vi "Calibrations_Save.vi"(8 "error in":errorcluster, 11 "Subsystem":string="MySubsystem") -> (0 "error out":errorcluster)   [LabVIEW 2020]
uses:
  <vilib>/Utility/config.llb/Write Key (I32).vi
  <vilib>/Rock Robotics/Network Tables/NT Write Number.vi
  <vilib>/Utility/config.llb/Write Key (Double).vi
  <vilib>/Rock Robotics/Network Tables/NT Write String.vi
  <vilib>/Utility/config.llb/Write Key (String).vi
  <vilib>/Utility/config.llb/Write Key (Boolean).vi
  <vilib>/Rock Robotics/Network Tables/NT Write Boolean.vi
  <vilib>/Utility/config.llb/NI_LVConfig.lvlib
  <vilib>/Utility/Data Type/NI_Data Type.lvlib
panel:
  # "The calling VI will need to include a reference for the subsystem Global.vi. If this is omitted, this VI will not\nbe able to resolve the reference to the VI to iterate through the front-panel controls.e"
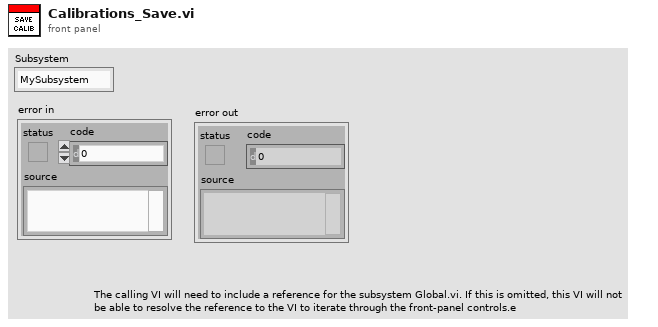
[diagram p1: front panel]
types:
  T1 = typedef "NI_LVConfig.lvlib/Config Data RefNum.ctl" = refnum<k1>
  T2 = typedef "NI_Data Type.lvlib/Data Type.ctl" = enum8{"Invalid Type", "Void", "I8", "I16", "I32", "I64", "U8", "U16", "U32", "U64", "Single Float", "Double Float", "Extended Float", "Single Complex", "Double Complex", "Extended Complex", "Enum U8", "Enum U16", "Enum U32", "Enum U64", "Single Float With Unit", "Double Float With Unit", "Extended Float With Unit", "Single Complex with Unit", "Double Complex with Unit", "Extended Complex with Unit", "Boolean", "String", "Path", "Picture", "Tag", "Array", "Cluster", "Variant", "LV Variant", "Waveform", "Timestamp", "Digital Waveform", "Digital Data", "ExpressData", "Refnum", "External Data", "VI", "Poly VI", "LabVIEW Class Instance", "Fixed Point", "Set Collection", "Map Collection"}
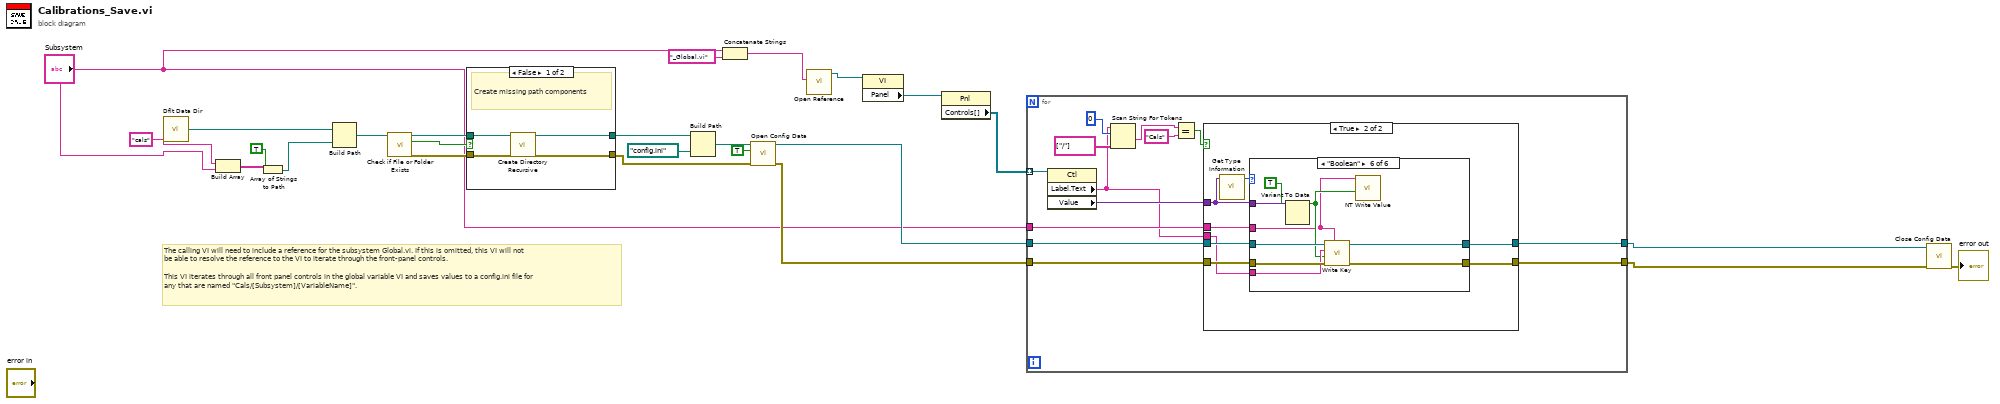
[diagram p0: block diagram]
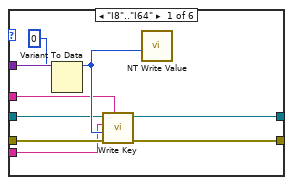
[diagram p3: hidden frame]
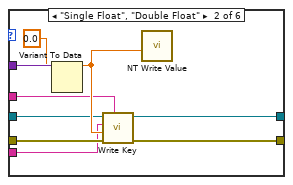
[diagram p4: hidden frame]
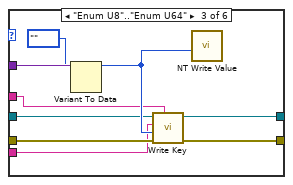
[diagram p5: hidden frame]
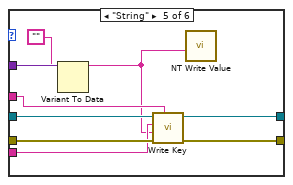
[diagram p7: hidden frame]
diagram:
  # "The calling VI will need to include a reference for the subsystem Global.vi. If this is omitted, this VI will not\nbe able to resolve the reference to the VI to iterate through the front-panel controls.\n\nThis VI iterates through all front panel controls in the global variable VI and saves values to a config.ini file for\nany that are named \"Cals/[Subsystem]/[VariableName]\"."
  n1 = call <vilib>:"Dflt Data Dir.vi"() -> ("App:Default Data Directory"=w25:path)
  n2 = Build Array("cals" ("string"), "Subsystem") -> (w4:string[])
  n3 = Array of Strings to Path(0:w4, 1:TRUE ("relative")) -> (2:w3:path)
  n4 = Build Path(base path=w25, name or relative path=w3) -> (appended path=w24:path)
  n5 = call <vilib>:"Check if File or Folder Exists.vi"("path"=w24) -> ("error out"=w21:errorcluster, "file or folder exists?"=w23:bool, "dup path"=w22:path)  [unwired: 8 in]
  n6 = case shown="False" w23 {
    tunnel: w22 -> [w29 w31]
    tunnel: w21 -> [w28 w30]
    tunnel: [w27 w31] -> w20
    tunnel: [w26 w30] -> w16
    frame False {
      # "Create missing path components"
      n7 = call <vilib>:"Create Directory Recursive.vi"("error in (no error)"=w28, "directory"=w29) -> ("error out"=w26:errorcluster, "directory copy"=w27:path)  [unwired: 3 in, 1 out]
    }
    frame True {
      # "Bypass"
    }
  }
  n8 = Build Path(base path=w20, name or relative path=path "config.ini") -> (appended path=w18:path)
  n9 = Concatenate Strings("Subsystem", "_Global.vi" ("string")) -> (w14:string)
  n10 = call <vilib>:"Open Config Data.vi"("error in (no error)"=w16, "create file if necessary (T)"=TRUE, "configuration file path"=w18) -> ("error out"=w7:errorcluster, "refnum"=w10:T1)  [unwired: 6 in, 1 out]
  n11 = call "Open Reference.vi"("Front Panel VI Name"=w14) -> ("Front Panel Reference"=w13:refnum<vi>)  [unwired: 5 in, 1 out]
  n12 = property class="VI"(reference=w13) -> ("Panel"=w12:refnum<vi>)  [unwired: 1 in, 2 out]
  n13 = property class="Pnl"(reference=w12) -> ("Controls[]"=w11:refnum<vi>[])  [unwired: 1 in, 2 out]
  n14 = for {
    tunnel: w11 -> [w44] mode=indexing
    tunnel: w10 -> [w42]
    tunnel: "Subsystem" -> [w41]
    tunnel: [w40] -> w9
    tunnel: [w39] -> w8
    tunnel: w7 -> [w38]
    n15 = property class="Ctl"(reference=w44) -> ("Label.Text"=w33:string, "Value"=w43:variant)  [unwired: 1 in, 2 out]
    n16 = Scan String For Tokens(6:string[] ["/"] ("operators (none)"), 8:0 ("offset"), 9:w33) -> (1:w32:string)  [unwired: 3 in, 3 out]
    n17 = Equal?(x=w32, y="Cals") -> (x = y?=w34:bool)
    n18 = case shown="True" w34 {
      tunnel: w43 -> [_ w53]
      tunnel: w42 -> [w46 w52]
      tunnel: w41 -> [_ w51]
      tunnel: [w46 w50] -> w40
      tunnel: [w45 w49] -> w39
      tunnel: w38 -> [w45 w48]
      tunnel: w33 -> [_ w47]
      frame False {
      }
      frame True {
        n19 = call <vilib>:"Get Type Information.vi"("variant"=w53) -> ("type"=w54:T2)  [unwired: 6 in, 4 out]
        n20 = case shown="\"Boolean\"" w54 {
          tunnel: w53 -> [w63 w72 w81 _ w86 w96]
          tunnel: w52 -> [w61 w70 w79 w83 w92 w101]
          tunnel: w51 -> [w60 w69 w78 _ w91 w93]
          tunnel: [w59 w68 w77 w83 w90 w100] -> w50
          tunnel: [w58 w67 w76 w82 w89 w99] -> w49
          tunnel: w48 -> [w57 w66 w75 w82 w88 w98]
          tunnel: w47 -> [w56 w65 w74 _ w87 w97]
          frame "I8".."I64" {
            n21 = Variant To Data(type=0, Variant=w63) -> (data=w62:i32)  [unwired: 1 in, 1 out]
            n22 = call-poly <vilib>:"Write Key.vi"("section"=w60, "error in (no error)"=w57, "value"=w62, "key"=w56, "refnum"=w61) -> ("error out"=w58:errorcluster, "refnum out"=w59:T1)  [unwired: 4 in, 1 out]
            n23 = call-poly <vilib>:"NT Write Value.vi"("Numeric"=w62) -> ()  [unwired: 10 in, 1 out]
          }
          frame "Single Float", "Double Float" {
            n24 = Variant To Data(type=0.0, Variant=w72) -> (data=w71:dbl)  [unwired: 1 in, 1 out]
            n25 = call-poly <vilib>:"Write Key.vi"("section"=w69, "error in (no error)"=w66, "value"=w71, "key"=w65, "refnum"=w70) -> ("error out"=w67:errorcluster, "refnum out"=w68:T1)  [unwired: 4 in, 1 out]
            n26 = call-poly <vilib>:"NT Write Value.vi"("Numeric"=w71) -> ()  [unwired: 10 in, 1 out]
          }
          frame "Enum U8".."Enum U64" {
            n27 = Variant To Data(type=enum16{""}."", Variant=w81) -> (data=w80:enum16{""})  [unwired: 1 in, 1 out]
            n28 = call-poly <vilib>:"Write Key.vi"("section"=w78, "error in (no error)"=w75, "value"=w80, "key"=w74, "refnum"=w79) -> ("error out"=w76:errorcluster, "refnum out"=w77:T1)  [unwired: 4 in, 1 out]
            n29 = call-poly <vilib>:"NT Write Value.vi"("Numeric"=w80) -> ()  [unwired: 10 in, 1 out]
          }
          frame Default {
          }
          frame "String" {
            n30 = Variant To Data(type="", Variant=w86) -> (data=w84:string)  [unwired: 1 in, 1 out]
            n31 = call-poly <vilib>:"Write Key.vi"("section"=w91, "error in (no error)"=w88, "value"=w84, "key"=w87, "refnum"=w92) -> ("error out"=w89:errorcluster, "refnum out"=w90:T1)  [unwired: 4 in, 1 out]
            n32 = call-poly <vilib>:"NT Write Value.vi"("String"=w84) -> ()  [unwired: 10 in, 1 out]
          }
          frame "Boolean" {
            n33 = Variant To Data(type=TRUE, Variant=w96) -> (data=w94:bool)  [unwired: 1 in, 1 out]
            n34 = call-poly <vilib>:"Write Key.vi"("section"=w93, "error in (no error)"=w98, "value"=w94, "key"=w97, "refnum"=w101) -> ("error out"=w99:errorcluster, "refnum out"=w100:T1)  [unwired: 4 in, 1 out]
            n35 = call-poly <vilib>:"NT Write Value.vi"("Boolean"=w94, "Name"=w93) -> ()  [unwired: 9 in, 1 out]
          }
        }
      }
    }
  }
  n36 = call <vilib>:"Close Config Data.vi"("error in (no error)"=w8, "refnum"=w9) -> ("error out"=→"error out":errorcluster)  [unwired: 8 in, 1 out]
